vi "Parse Error.vi"(8 "error in (no error)":errorcluster, 10 "error code":i32, 11 "body in":string) -> (0 "error out":errorcluster, 3 "body out":string, 4 "error data":string[](array[string]))   [LabVIEW 2014, in "Random JSON API.lvlib"]
uses:
  Random JSON API.lvlib
  <vilib>/Utility/error.llb/DialogType.ctl
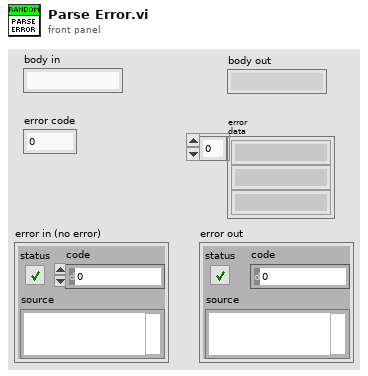
[diagram p1: front panel]
types:
  T1 = typedef "DialogType.ctl" = u16
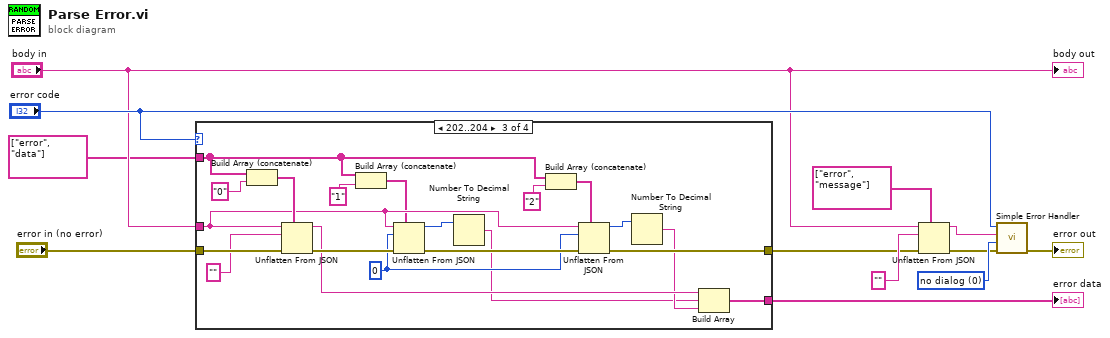
[diagram p0: block diagram]
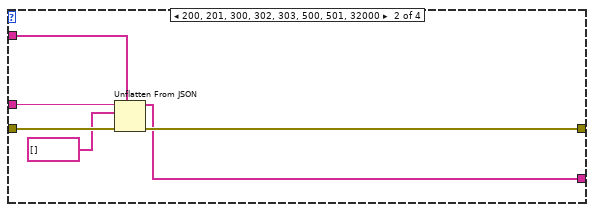
[diagram p3: hidden frame]
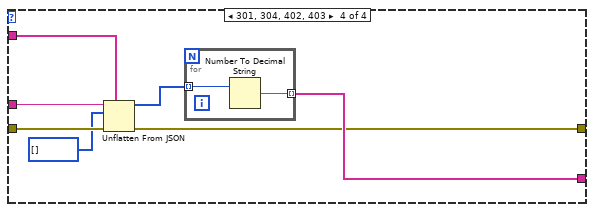
[diagram p4: hidden frame]
diagram:
  w11 = T1 0 items=["no dialog", "OK message", "continue or stop message", "OK message + warnings", "continue/stop + warnings"] ("type of dialog (OK msg:1)")
  n1 = case shown="202..204" "error code" {
    tunnel: "error in (no error)" -> [w13 w19 w39 w46]
    tunnel: "body in" -> [_ w17 w32 w45]
    tunnel: [w13 w18 w33 w40] -> w3
    tunnel: string[] ["error", "data"] ("path") -> [_ w16 w31 w44]
    tunnel: [_ w14 w24 w41] -> w1
    frame Default {
    }
    frame 200, 201, 300, 302, 303, 500, 501, 32000 {
      n2 = Unflatten From JSON(path=w16, JSON string=w17, type and defaults=string[] [], error in (no error)=w19) -> (value=w14:string[], error out=w18:errorcluster)  [unwired: 3 in]
    }
    frame 202..204 {
      w26 = 0
      n3 = Build Array (concatenate)(w31, "0") -> (w37:string[])
      n4 = Unflatten From JSON(path=w37, JSON string=w32, type and defaults="", error in (no error)=w39) -> (value=w25:string, error out=w35:errorcluster)  [unwired: 3 in]
      n5 = Build Array (concatenate)(w31, "1") -> (w27:string[])
      n6 = Unflatten From JSON(path=w27, JSON string=w32, type and defaults=w26, error in (no error)=w35) -> (value=w21:i32, error out=w34:errorcluster)  [unwired: 3 in]
      n7 = Number To Decimal String(number=w21) -> (decimal integer string=w20:string)  [unwired: 1 in]
      n8 = Build Array (concatenate)(w31, "2") -> (w28:string[])
      n9 = Unflatten From JSON(path=w28, JSON string=w32, type and defaults=w26, error in (no error)=w34) -> (value=w23:i32, error out=w33:errorcluster)  [unwired: 3 in]
      n10 = Number To Decimal String(number=w23) -> (decimal integer string=w22:string)  [unwired: 1 in]
      n11 = Build Array(w25, w20, w22) -> (w24:string[])
    }
    frame 301, 304, 402, 403 {
      n12 = Unflatten From JSON(path=w44, JSON string=w45, type and defaults=i32[] [], error in (no error)=w46) -> (value=w42:i32[], error out=w40:errorcluster)  [unwired: 3 in]
      n13 = for {
        tunnel: w42 -> [w48] mode=indexing
        tunnel: [w47] -> w41 mode=indexing
        n14 = Number To Decimal String(number=w48) -> (decimal integer string=w47:string)  [unwired: 1 in]
      }
    }
  }
  "error data" <- w1
  n15 = Unflatten From JSON(path=string[] ["error", "message"], JSON string="body in", type and defaults="", error in (no error)=w3) -> (value=w10:string, error out=w9:errorcluster)  [unwired: 3 in]
  n16 = call <vilib>:"Simple Error Handler.vi"("error code (no error:0)"="error code", "error source (\" \")"=w10, "type of dialog (OK msg:1)"=w11, "error in (no error)"=w9) -> ("error out"=→"error out":errorcluster)  [unwired: 1 in, 4 out]
  "body out" <- "body in"
